vi "set_Thre.vi"(8 "错误输入（无错误）":errorcluster, 9 "命令":u8 max=63 step=1, 10 "数字":u16=49152, 11 "VISA资源名称":refnum<visa-resource-name>) -> (0 "错误输出":errorcluster, 3 "VISA资源名称输出":refnum<visa-resource-name>)   [LabVIEW 2014]
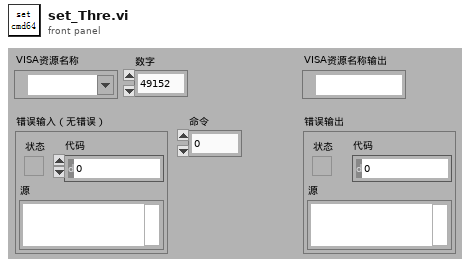
[diagram p1: front panel]
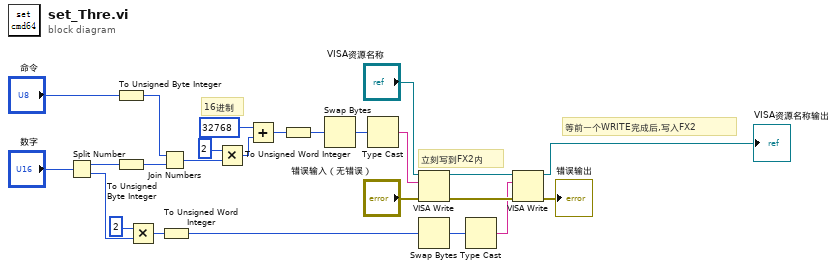
[diagram p0: block diagram]
diagram:
  # "等前一个WRITE完成后,写入FX2"
  # "立刻写到FX2内"
  # "16进制"
  n1 = Split Number(x="数字") -> (hi(x)=w6:u8, lo(x)=w11:u8)
  n2 = To Unsigned Byte Integer(number="命令") -> (unsigned 8bit integer=w8:u8)
  n3 = To Unsigned Byte Integer(number=w6) -> (unsigned 8bit integer=w7:u8)
  n4 = Multiply(x=u64 2, y=w11) -> (x*y=w2:u64)
  n5 = Join Numbers(hi=w8, lo=w7) -> ((hi.lo)=w16:u16)
  n6 = To Unsigned Word Integer(number=w2) -> (unsigned 16bit integer=w3:u16)
  n7 = Multiply(x=u64 2, y=w16) -> (x*y=w14:u64)
  n8 = Add(x=32768 ("数字"), y=w14) -> (x+y=w5:u64)
  n9 = To Unsigned Word Integer(number=w5) -> (unsigned 16bit integer=w4:u16)
  n10 = Swap Bytes(anything=w4) -> (byte swapped=w23:u16)
  n11 = Type Cast(x=w23) -> (*(type *) &x=w22:string)  [unwired: 1 in]
  n12 = VISA Write(VISA resource name="VISA资源名称", write buffer=w22, error in (no error)="错误输入（无错误）") -> (VISA resource name out=w21:refnum<visa-resource-name>, error out=w19:errorcluster)  [unwired: 1 out]
  n13 = Swap Bytes(anything=w3) -> (byte swapped=w10:u16)
  n14 = Type Cast(x=w10) -> (*(type *) &x=w9:string)  [unwired: 1 in]
  n15 = VISA Write(VISA resource name=w21, write buffer=w9, error in (no error)=w19) -> (VISA resource name out=→"VISA资源名称输出":refnum<visa-resource-name>, error out=→"错误输出":errorcluster)  [unwired: 1 out]
